vi "ObslugaPieca.vi"() -> ()   [LabVIEW 2012]
doc: "Use this template to build a user interface event handler design pattern. Use this pattern for dialog boxes and other user interfaces. You also can create and execute user-defined events that the VI can handle the same way as user interface events."
uses:
  MachineStatesEnum.ctl
  <vilib>/Utility/file.llb/Write To Spreadsheet File (I64).vi
  <vilib>/Utility/file.llb/Write To Spreadsheet File (string).vi
  <vilib>/Utility/file.llb/Read From Spreadsheet File (string).vi
panel:
  out "wyniki":i16[](array[numeric])
  in  "doStop":bool
  out "Data loaded":bool=TRUE
  in  "SendTelegramDone":bool=TRUE
  in  "Next state":T1=enum."Initialized"
  in  "ProgramStopped":bool=TRUE
  out "Telegrams array":string[](array[string])
  in  "Tab Control":T2(tab)
  in  "Initialize":bool
  in  "VISA resource name":refnum<visa-resource-name>="COM10"
  in  "Load configuration":bool
  in  "Save configuration":bool
  in  "Configure":bool
  out "Telegram1":string
  in  "Temperatura 1":u16 max=400 step=1 format="%03d"
  in  "Godzin 1":u16 max=24 step=1 format="%02d"
  in  "Minut 1":u16 max=59 step=1 format="%02d"
  in  "Sekund 1":u16 max=59 step=1 format="%02d"
  out "Telegram2":string
  in  "Temperatura 2":u16 max=400 step=1 format="%03d"
  in  "Godzin 2":u16 max=24 step=1 format="%02d"
  in  "Minut 2":u16 max=59 step=1 format="%02d"
  in  "Sekund 2":u16 max=59 step=1 format="%02d"
  out "Telegram3":string
  in  "Temperatura 3":u16 max=400 step=1 format="%03d"
  in  "Godzin 3":u16 max=24 step=1 format="%02d"
  in  "Minut 3":u16 max=59 step=1 format="%02d"
  in  "Sekund 3":u16 max=59 step=1 format="%02d"
  in  "Temperatura 6":u16 max=400 step=1 format="%03d"
  in  "Godzin 6":u16 max=24 step=1 format="%02d"
  in  "Minut 6":u16 max=59 step=1 format="%02d"
  in  "Sekund 6":u16 max=59 step=1 format="%02d"
  out "Telegram4":string
  in  "Temperatura 4":u16 max=400 step=1 format="%03d"
  in  "Godzin 4":u16 max=24 step=1 format="%02d"
  in  "Minut 4":u16 max=59 step=1 format="%02d"
  in  "Sekund 4":u16 max=59 step=1 format="%02d"
  in  "Temperatura 5":u16 max=400 step=1 format="%03d"
  in  "Godzin 5":u16 max=24 step=1 format="%02d"
  in  "Minut 5":u16 max=59 step=1 format="%02d"
  in  "Sekund 5":u16 max=59 step=1 format="%02d"
  out "Telegram6":string
  out "Telegram5":string
  out "Wykres zmian temperatury":i16[](graph)
  out "Stan pieca":string
  out "Numer  zadanego programu":string
  in  "Stop":bool
  in  "Port Errors":errorcluster
  out "OdpowiedŸ pieca":string
  in  "Odbiorcy":string
  in  "Wyœlij e-mail przy koñcu":bool
  # "Kolejne programy (nie obowi¹zkowe)"
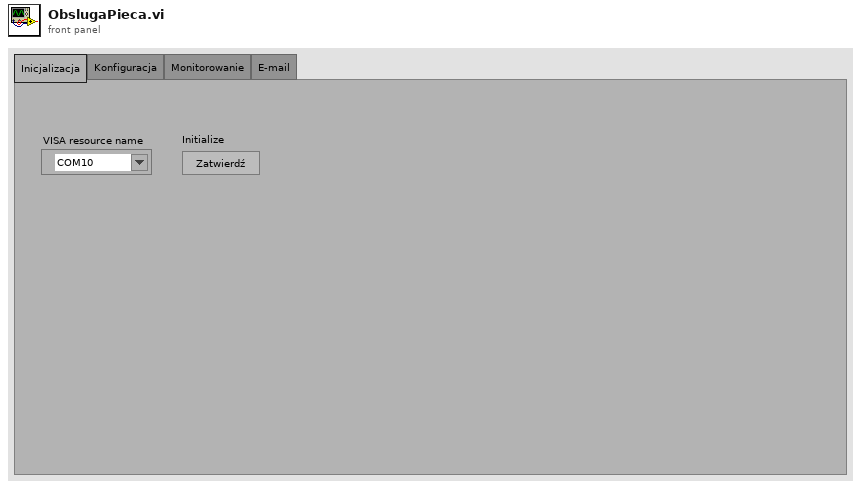
[diagram p1: front panel]
types:
  T1 = typedef "MachineStatesEnum.ctl" = enum16{"StartState", "Initialized", "Configured", "Monitoring", "Ended", "Stopped", "ErrorState"}
  T2 = enum32{"Inicjalizacja", "Konfiguracja", "Monitorowanie", "E-mail"}
  T3 = enum32{"Inicjalizacja", "Konfiguracja", "Monitorowanie"}
  T4 = enum8{"Enabled", "Disabled", "Disabled and Grayed Out"}
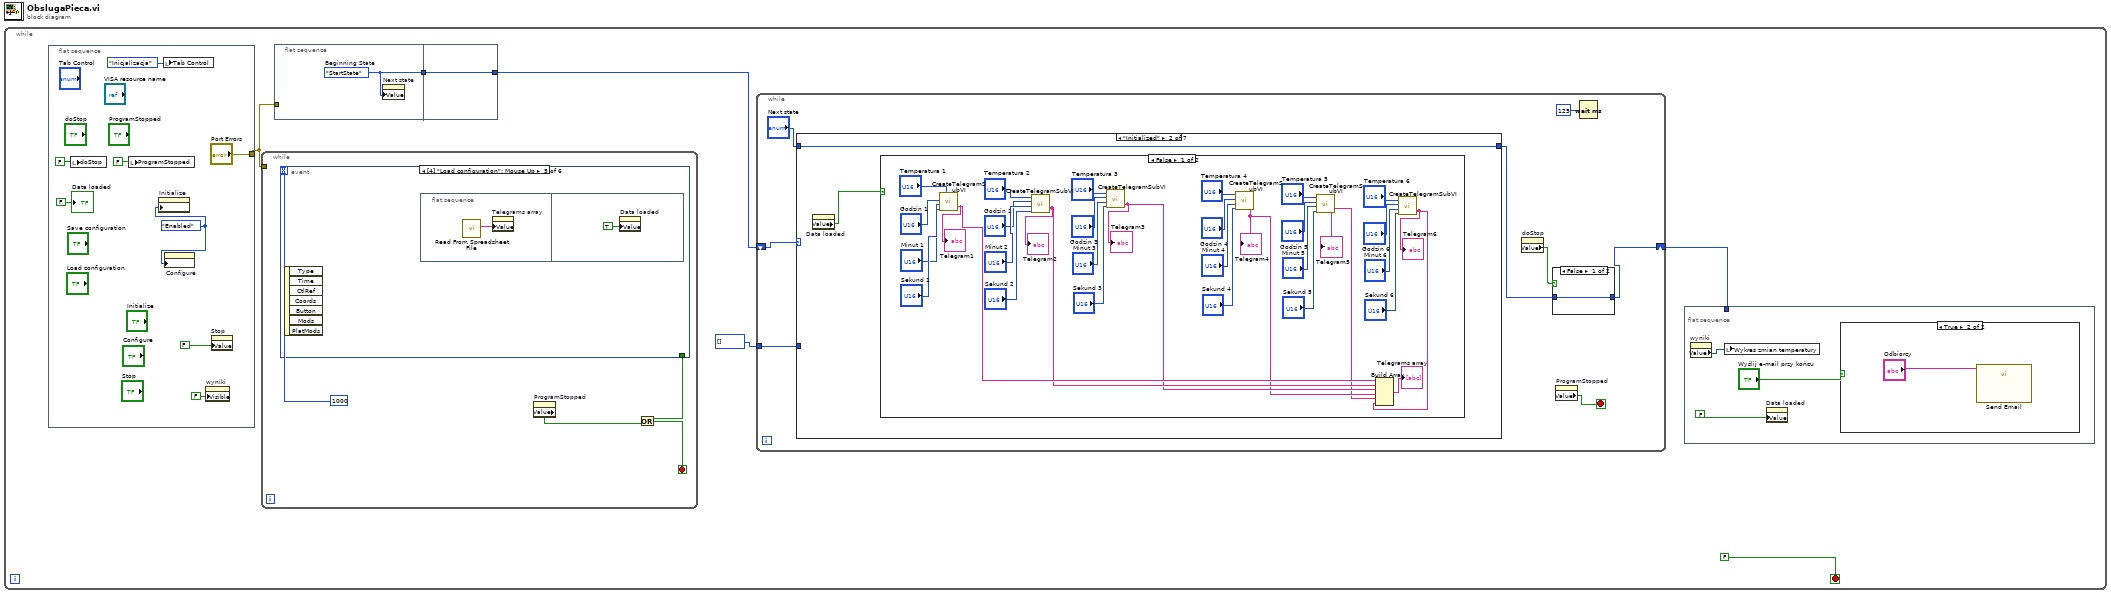
[diagram p0: block diagram]
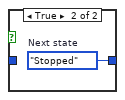
[diagram p3: hidden frame]
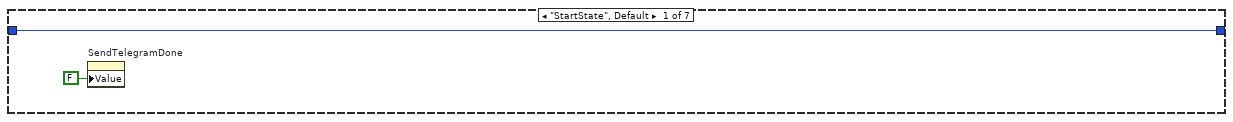
[diagram p4: hidden frame]
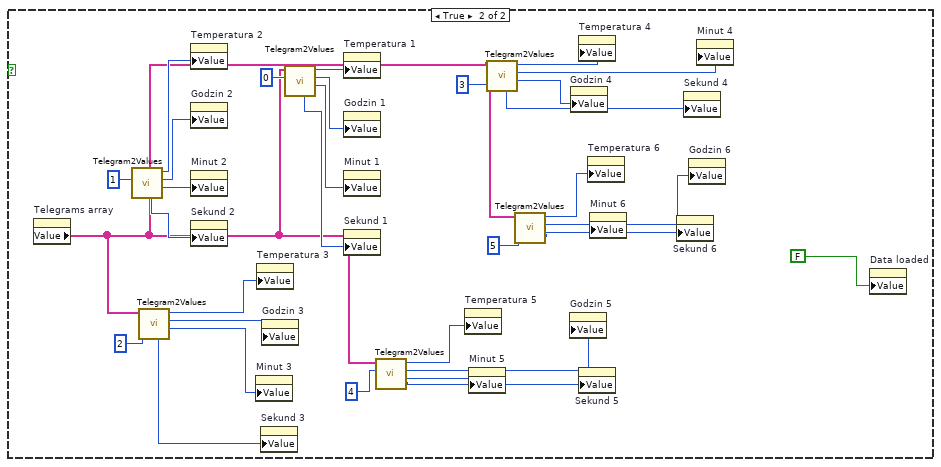
[diagram p5: hidden frame]
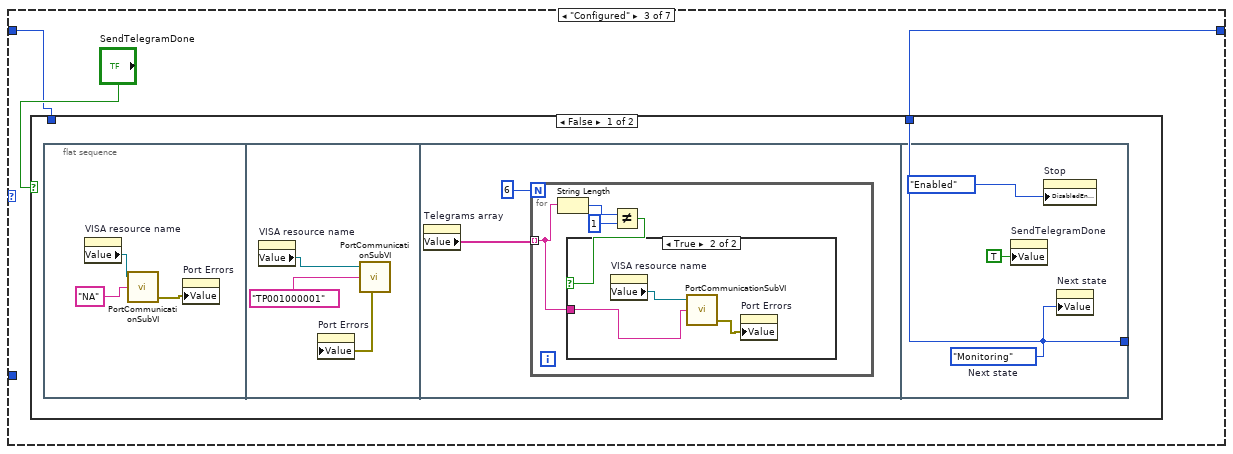
[diagram p6: hidden frame]
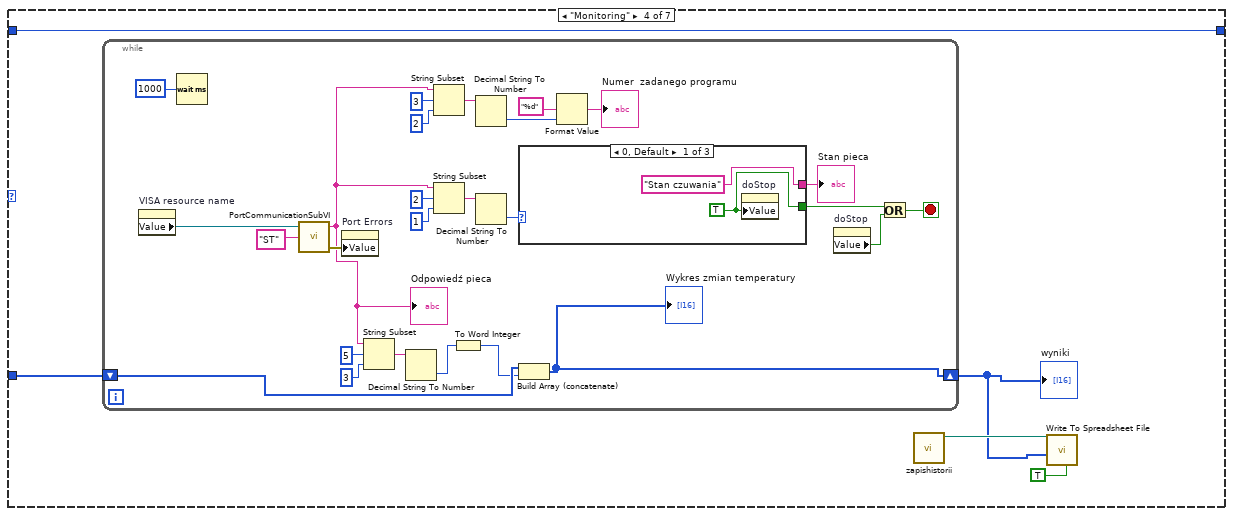
[diagram p9: hidden frame]
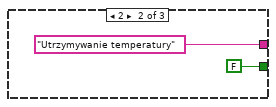
[diagram p10: hidden frame]
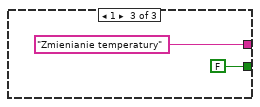
[diagram p11: hidden frame]
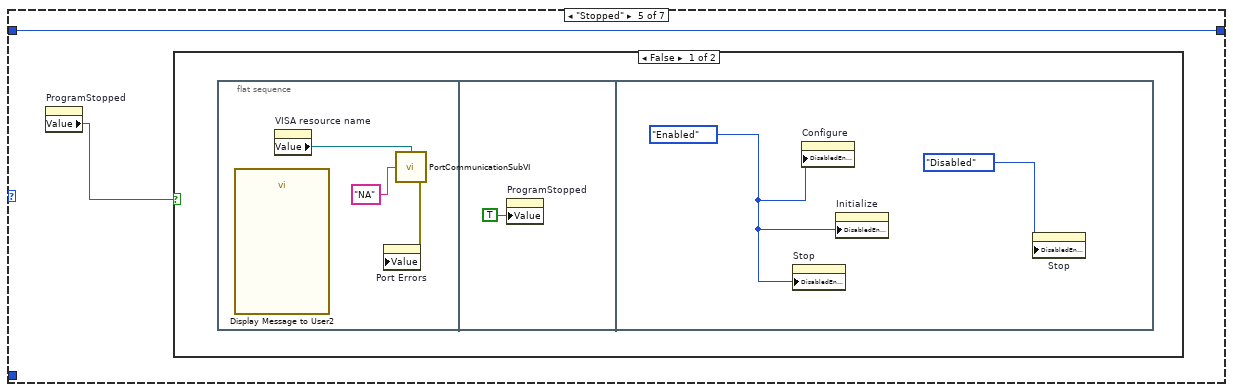
[diagram p12: hidden frame]
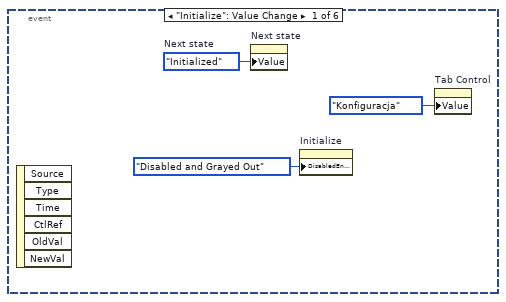
[diagram p16: hidden frame]
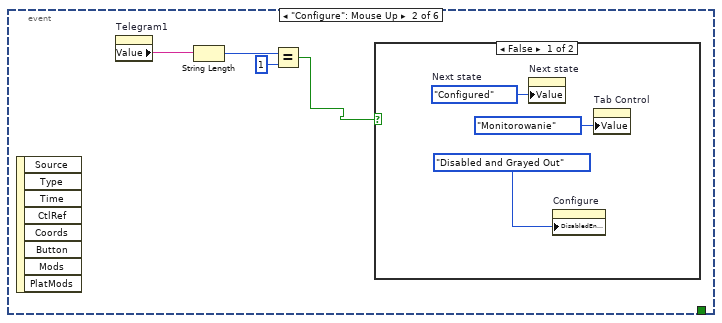
[diagram p17: hidden frame]
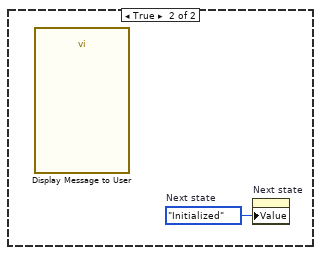
[diagram p18: hidden frame]
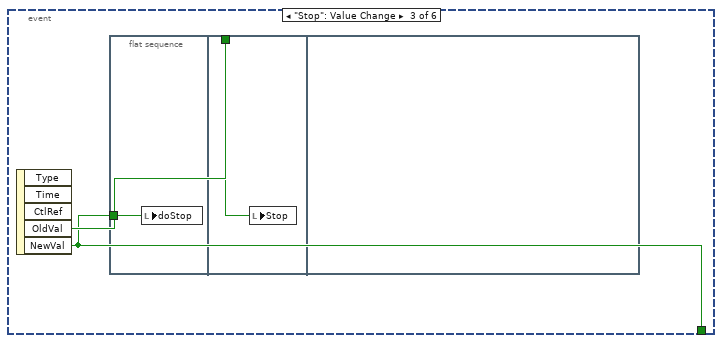
[diagram p19: hidden frame]
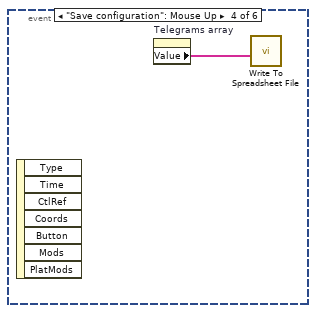
[diagram p20: hidden frame]
diagram:
  n1 = while {
    stop <- FALSE stop-if-true
    n2 = flat-sequence {
      tunnel: ["Port Errors"] -> w4
      frame #0 {
        w13 = T4."Enabled" ("Disabled")
        n3 = local write "doStop"(FALSE ("doStop")) -> ()
        n4 = local write "ProgramStopped"(FALSE ("ProgramStopped")) -> ()
        n5 = property on="Initialize" class="Bool"("DisabledEnum"=w13) -> ()  [unwired: 2 in, 2 out]
        n6 = local write "Tab Control"(T3."Inicjalizacja" ("Tab Control")) -> ()
        n7 = property on="Configure" class="Bool"("DisabledEnum"=w13) -> ()  [unwired: 2 in, 2 out]
        n8 = property on="wyniki" class="Arr (strict)"("Visible"=FALSE) -> ()  [unwired: 2 in, 2 out]
        n9 = property on="Stop" class="Bool (strict)"("Value"=FALSE) -> ()  [unwired: 2 in, 2 out]
        "Data loaded" <- FALSE ("Data loaded")
      }
    }
    n10 = while {
      tunnel: w4 -> [_]
      stop <- w169 stop-if-true
      n11 = event shown="[4] \"Load configuration\": Mouse Up" {
        selector: _ -> [_ _ _ _ _ _]
        dyn-events: _ -> [_ _ _ _ _ _]
        timeout: 1000 -> [_ _ _ _ _ _]
        tunnel: [_ _ w183 _ _ _] -> w171
        event "Initialize": Value Change {
          w173 = MachineStatesEnum."Initialized"  # Next state
          n12 = event-data() -> ()  [unwired: 1 in, 6 out]
          n13 = property on="Next state" class="Enum (strict)"("Value"=w173) -> ()  [unwired: 2 in, 2 out]
          n14 = property on="Initialize" class="Bool"("DisabledEnum"=T4."Disabled and Grayed Out" ("Disabled")) -> ()  [unwired: 2 in, 2 out]
          n15 = property on="Tab Control" class="TabCtl (strict)"("Value"=T3."Konfiguracja" ("Tab Control")) -> ()  [unwired: 2 in, 2 out]
        }
        event "Configure": Mouse Up {
          n16 = event-data() -> ()  [unwired: 1 in, 8 out]
          n17 = property on="Telegram1" class="Str"() -> ("Value"=w176:string)  [unwired: 2 in, 2 out]
          n18 = String Length(string=w176) -> (length=w178:i32)
          n19 = Equal?(x=w178, y=1) -> (x = y?=w175:bool)
          n20 = case shown="False" w175 {
            frame False {
              w180 = MachineStatesEnum."Configured"  # Next state
              n21 = property on="Next state" class="Enum (strict)"("Value"=w180) -> ()  [unwired: 2 in, 2 out]
              n22 = property on="Configure" class="Bool"("DisabledEnum"=T4."Disabled and Grayed Out" ("Disabled")) -> ()  [unwired: 2 in, 2 out]
              n23 = property on="Tab Control" class="TabCtl (strict)"("Value"=T3."Monitorowanie" ("Tab Control")) -> ()  [unwired: 2 in, 2 out]
            }
            frame True {
              w182 = MachineStatesEnum."Initialized"  # Next state
              n24 = call "Display Message to User"() -> ()  [unwired: 10 in, 2 out]
              n25 = property on="Next state" class="Enum (strict)"("Value"=w182) -> ()  [unwired: 2 in, 2 out]
            }
          }
        }
        event "Stop": Value Change {
          n26 = event-data() -> ("OldVal"=w184:bool, "NewVal"=w183:bool)  [unwired: 1 in, 3 out]
          n27 = flat-sequence {
            tunnel: w183 -> [w185]
            tunnel: w184 -> [w186]
            frame #0 {
              n28 = local write "doStop"(w185) -> ()
            }
            frame #1 {
              n29 = local write "Stop"(w186) -> ()
            }
            frame #2 {
            }
          }
        }
        event "Save configuration": Mouse Up {
          n30 = event-data() -> ()  [unwired: 1 in, 7 out]
          n31 = property on="Telegrams array" class="Arr (strict)"() -> ("Value"=w187:string[])  [unwired: 2 in, 2 out]
          n32 = call-poly <vilib>:"Write To Spreadsheet File.vi"("1D data"=w187) -> ()  [unwired: 7 in, 1 out]
        }
        event "Load configuration": Mouse Up {
          n33 = event-data() -> ()  [unwired: 1 in, 7 out]
          n34 = flat-sequence {
            frame #0 {
              n35 = call-poly <vilib>:"Read From Spreadsheet File.vi"() -> ("first row"=w188:string[])  [unwired: 7 in, 4 out]
              n36 = property on="Telegrams array" class="Arr (strict)"("Value"=w188) -> ()  [unwired: 2 in, 2 out]
            }
            frame #1 {
              n37 = property on="Data loaded" class="Bool (strict)"("Value"=TRUE) -> ()  [unwired: 2 in, 2 out]
            }
          }
        }
        event Timeout {
          n38 = event-data() -> ()  [unwired: 1 in, 3 out]
        }
      }
      n39 = property on="ProgramStopped" class="Bool (strict)"() -> ("Value"=w170:bool)  [unwired: 2 in, 2 out]
      n40 = Or(x=w171, y=w170) -> (x .or. y?=w169:bool)
    }
    n41 = flat-sequence {
      tunnel: [w19] -> w6
      tunnel: w4 -> [_]
      tunnel: [w20] -> w5
      tunnel: w6 -> [w20]
      frame #0 {
        w19 = MachineStatesEnum."StartState"  # Beginning State
        n42 = property on="Next state" class="Enum (strict)"("Value"=w19) -> ()  [unwired: 2 in, 2 out]
      }
      frame #1 {
      }
    }
    n43 = while {
      shift-right: [w23] -> w2
      shift-left: w5 -> [w27]
      tunnel: i16[] [] -> [w21]
      stop <- w25 stop-if-true
      n44 = case shown="\"Initialized\"" w27 {
        selector: w27 -> [_ _ _ _ _ w166 w167]
        tunnel: [w32 w34 w98 w125 w159 w166 w167] -> w24
        tunnel: "Next state" -> [w32 w34 w99 w125 w159 _ _]
        tunnel: w21 -> [_ _ _ w124 _ _ _]
        frame "StartState", Default {
          n45 = property on="SendTelegramDone" class="Bool (strict)"("Value"=FALSE ("SendTelegramDone")) -> ()  [unwired: 2 in, 2 out]
        }
        frame "Initialized" {
          n46 = property on="Data loaded" class="Bool (strict)"() -> ("Value"=w33:bool)  [unwired: 2 in, 2 out]
          n47 = case shown="False" w33 {
            frame False {
              n48 = call "CreateTelegramSubVI.vi"("seconds"="Sekund 1", "minutes"="Minut 1", "hours"="Godzin 1", "temperature"="Temperatura 1") -> ("tempTelegram"=w41:string)  [unwired: 1 in]
              "Telegram1" <- w41
              n49 = call "CreateTelegramSubVI.vi"("seconds"="Sekund 2", "minutes"="Minut 2", "hours"="Godzin 2", "temperature"="Temperatura 2") -> ("tempTelegram"=w40:string)  [unwired: 1 in]
              "Telegram2" <- w40
              n50 = call "CreateTelegramSubVI.vi"("seconds"="Sekund 3", "minutes"="Minut 3", "hours"="Godzin 3", "temperature"="Temperatura 3") -> ("tempTelegram"=w39:string)  [unwired: 1 in]
              "Telegram3" <- w39
              n51 = call "CreateTelegramSubVI.vi"("seconds"="Sekund 4", "minutes"="Minut 4", "hours"="Godzin 4", "temperature"="Temperatura 4") -> ("tempTelegram"=w38:string)  [unwired: 1 in]
              "Telegram4" <- w38
              n52 = call "CreateTelegramSubVI.vi"("seconds"="Sekund 5", "minutes"="Minut 5", "hours"="Godzin 5", "temperature"="Temperatura 5") -> ("tempTelegram"=w37:string)  [unwired: 1 in]
              "Telegram5" <- w37
              n53 = call "CreateTelegramSubVI.vi"("seconds"="Sekund 6", "minutes"="Minut 6", "hours"="Godzin 6", "temperature"="Temperatura 6") -> ("tempTelegram"=w36:string)  [unwired: 1 in]
              "Telegram6" <- w36
              n54 = Build Array(w41, w40, w39, w38, w37, w36) -> (→"Telegrams array":string[])
            }
            frame True {
              n55 = property on="Telegrams array" class="Arr (strict)"() -> ("Value"=w87:string[])  [unwired: 2 in, 2 out]
              n56 = call "Telegram2Values.vi"("index"=1, "Value"=w87) -> ("Numeric 2"=w89:u16, "Numeric 3"=w90:u16, "Numeric 4"=w91:u16, "Numeric"=w88:u16)  [unwired: 6 in]
              n57 = call "Telegram2Values.vi"("index"=2, "Value"=w87) -> ("Numeric 2"=w80:u16, "Numeric 3"=w81:u16, "Numeric 4"=w82:u16, "Numeric"=w79:u16)  [unwired: 6 in]
              n58 = property on="Temperatura 2" class="DigNum (strict)"("Value"=w91) -> ()  [unwired: 2 in, 2 out]
              n59 = property on="Godzin 2" class="DigNum (strict)"("Value"=w90) -> ()  [unwired: 2 in, 2 out]
              n60 = property on="Minut 2" class="DigNum (strict)"("Value"=w89) -> ()  [unwired: 2 in, 2 out]
              n61 = property on="Sekund 2" class="DigNum (strict)"("Value"=w88) -> ()  [unwired: 2 in, 2 out]
              n62 = property on="Minut 3" class="DigNum (strict)"("Value"=w80) -> ()  [unwired: 2 in, 2 out]
              n63 = property on="Temperatura 3" class="DigNum (strict)"("Value"=w82) -> ()  [unwired: 2 in, 2 out]
              n64 = property on="Sekund 3" class="DigNum (strict)"("Value"=w79) -> ()  [unwired: 2 in, 2 out]
              n65 = property on="Godzin 3" class="DigNum (strict)"("Value"=w81) -> ()  [unwired: 2 in, 2 out]
              n66 = call "Telegram2Values.vi"("index"=0, "Value"=w87) -> ("Numeric 2"=w94:u16, "Numeric 3"=w96:u16, "Numeric 4"=w97:u16, "Numeric"=w93:u16)  [unwired: 6 in]
              n67 = property on="Temperatura 1" class="DigNum (strict)"("Value"=w97) -> ()  [unwired: 2 in, 2 out]
              n68 = property on="Godzin 1" class="DigNum (strict)"("Value"=w96) -> ()  [unwired: 2 in, 2 out]
              n69 = property on="Minut 1" class="DigNum (strict)"("Value"=w94) -> ()  [unwired: 2 in, 2 out]
              n70 = property on="Sekund 1" class="DigNum (strict)"("Value"=w93) -> ()  [unwired: 2 in, 2 out]
              n71 = call "Telegram2Values.vi"("index"=4, "Value"=w87) -> ("Numeric 2"=w72:u16, "Numeric 3"=w73:u16, "Numeric 4"=w74:u16, "Numeric"=w71:u16)  [unwired: 6 in]
              n72 = property on="Temperatura 5" class="DigNum (strict)"("Value"=w74) -> ()  [unwired: 2 in, 2 out]
              n73 = property on="Minut 5" class="DigNum (strict)"("Value"=w72) -> ()  [unwired: 2 in, 2 out]
              n74 = call "Telegram2Values.vi"("index"=3, "Value"=w87) -> ("Numeric 2"=w76:u16, "Numeric 3"=w77:u16, "Numeric 4"=w78:u16, "Numeric"=w75:u16)  [unwired: 6 in]
              n75 = call "Telegram2Values.vi"("index"=5, "Value"=w87) -> ("Numeric 2"=w68:u16, "Numeric 3"=w69:u16, "Numeric 4"=w70:u16, "Numeric"=w67:u16)  [unwired: 6 in]
              n76 = property on="Godzin 5" class="DigNum (strict)"("Value"=w73) -> ()  [unwired: 2 in, 2 out]
              n77 = property on="Godzin 4" class="DigNum (strict)"("Value"=w76) -> ()  [unwired: 2 in, 2 out]
              n78 = property on="Temperatura 4" class="DigNum (strict)"("Value"=w78) -> ()  [unwired: 2 in, 2 out]
              n79 = property on="Sekund 5" class="DigNum (strict)"("Value"=w71) -> ()  [unwired: 2 in, 2 out]
              n80 = property on="Temperatura 6" class="DigNum (strict)"("Value"=w70) -> ()  [unwired: 2 in, 2 out]
              n81 = property on="Minut 6" class="DigNum (strict)"("Value"=w68) -> ()  [unwired: 2 in, 2 out]
              n82 = property on="Sekund 6" class="DigNum (strict)"("Value"=w67) -> ()  [unwired: 2 in, 2 out]
              n83 = property on="Sekund 4" class="DigNum (strict)"("Value"=w75) -> ()  [unwired: 2 in, 2 out]
              n84 = property on="Godzin 6" class="DigNum (strict)"("Value"=w69) -> ()  [unwired: 2 in, 2 out]
              n85 = property on="Minut 4" class="DigNum (strict)"("Value"=w77) -> ()  [unwired: 2 in, 2 out]
              n86 = property on="Data loaded" class="Bool (strict)"("Value"=FALSE) -> ()  [unwired: 2 in, 2 out]
            }
          }
        }
        frame "Configured" {
          n87 = case shown="False" "SendTelegramDone" {
            tunnel: w99 -> [_ w120]
            tunnel: [w101 w120] -> w98
            frame False {
              n88 = flat-sequence {
                tunnel: [w118] -> w101
                frame #0 {
                  n89 = property on="VISA resource name" class="VISAName"() -> ("Value"=w102:refnum<visa-resource-name>)  [unwired: 2 in, 2 out]
                  n90 = call "PortCommunicationSubVI.vi"("Value"="NA", "VISA Refnum in"=w102) -> ("error out"=w103:errorcluster)  [unwired: 2 in, 1 out]
                  n91 = property on="Port Errors" class="Clust (strict)"("Value"=w103) -> ()  [unwired: 2 in, 2 out]
                }
                frame #1 {
                  n92 = property on="VISA resource name" class="VISAName"() -> ("Value"=w107:refnum<visa-resource-name>)  [unwired: 2 in, 2 out]
                  n93 = call "PortCommunicationSubVI.vi"("Value"="TP001000001", "VISA Refnum in"=w107) -> ("error out"=w106:errorcluster)  [unwired: 2 in, 1 out]
                  n94 = property on="Port Errors" class="Clust (strict)"("Value"=w106) -> ()  [unwired: 2 in, 2 out]
                }
                frame #2 {
                  n95 = property on="Telegrams array" class="Arr (strict)"() -> ("Value"=w108:string[])  [unwired: 2 in, 2 out]
                  n96 = for {
                    N: 6 -> [_]
                    tunnel: w108 -> [w110] mode=indexing
                    n97 = String Length(string=w110) -> (length=w111:i32)
                    n98 = Not Equal?(x=w111, y=1) -> (x != y?=w113:bool)
                    n99 = case shown="True" w113 {
                      tunnel: w110 -> [_ w115]
                      frame False {
                      }
                      frame True {
                        n100 = property on="VISA resource name" class="VISAName"() -> ("Value"=w116:refnum<visa-resource-name>)  [unwired: 2 in, 2 out]
                        n101 = call "PortCommunicationSubVI.vi"("Value"=w115, "VISA Refnum in"=w116) -> ("error out"=w114:errorcluster)  [unwired: 2 in, 1 out]
                        n102 = property on="Port Errors" class="Clust (strict)"("Value"=w114) -> ()  [unwired: 2 in, 2 out]
                      }
                    }
                  }
                }
                frame #3 {
                  w118 = MachineStatesEnum."Monitoring"  # Next state
                  n103 = property on="SendTelegramDone" class="Bool (strict)"("Value"=TRUE ("SendTelegramDone")) -> ()  [unwired: 2 in, 2 out]
                  n104 = property on="Stop" class="Bool (strict)"("DisabledEnum"=T4."Enabled" ("Disabled")) -> ()  [unwired: 2 in, 2 out]
                  n105 = property on="Next state" class="Enum (strict)"("Value"=w118) -> ()  [unwired: 2 in, 2 out]
                }
              }
            }
            frame True {
            }
          }
        }
        frame "Monitoring" {
          n106 = while {
            shift-right: [w126] -> w122
            shift-left: w124 -> [w129]
            stop <- w132 stop-if-true
            n107 = property on="VISA resource name" class="VISAName"() -> ("Value"=w137:refnum<visa-resource-name>)  [unwired: 2 in, 2 out]
            n108 = Wait (ms)(milliseconds to wait=u32 1000) -> ()  [unwired: 1 out]
            n109 = call "PortCommunicationSubVI.vi"("Value"="ST", "VISA Refnum in"=w137) -> ("error out"=w135:errorcluster, "read buffer"=w134:string)  [unwired: 2 in]
            "OdpowiedŸ pieca" <- w134
            n110 = property on="Port Errors" class="Clust (strict)"("Value"=w135) -> ()  [unwired: 2 in, 2 out]
            n111 = String Subset(string=w134, offset (0)=5, length (rest)=3 ("length (rest)")) -> (substring=w148:string)
            n112 = Decimal String To Number(string=w148) -> (number=w128:i32)  [unwired: 2 in, 1 out]
            n113 = String Subset(string=w134, offset (0)=3, length (rest)=2 ("length (rest)")) -> (substring=w140:string)
            n114 = String Subset(string=w134, offset (0)=2, length (rest)=1 ("length (rest)")) -> (substring=w145:string)
            n115 = To Word Integer(number=w128) -> (16bit integer=w127:i16)
            n116 = Decimal String To Number(string=w140) -> (number=w131:i32)  [unwired: 2 in, 1 out]
            n117 = Decimal String To Number(string=w145) -> (number=w143:i32)  [unwired: 2 in, 1 out]
            n118 = case shown="0, Default" w143 {
              tunnel: ["Stan czuwania" ("Stan pieca") "Utrzymywanie temperatury" ("Stan pieca") "Zmienianie temperatury" ("Stan pieca")] -> w144
              tunnel: [w152 FALSE ("y") FALSE ("y")] -> w133
              frame 0, Default {
                w152 = TRUE ("y")
                n119 = property on="doStop" class="Bool (strict)"("Value"=w152) -> ()  [unwired: 2 in, 2 out]
              }
              frame 2 {
              }
              frame 1 {
              }
            }
            "Stan pieca" <- w144
            n120 = Build Array (concatenate)(w129, w127) -> (w126:i16[])
            "Wykres zmian temperatury" <- w126
            n121 = Format Value(format string="%d", value (0)=w131) -> (output string=→"Numer  zadanego programu":string)  [unwired: 1 in]
            n122 = property on="doStop" class="Bool (strict)"() -> ("Value"=w130:bool)  [unwired: 2 in, 2 out]
            n123 = Or(x=w133, y=w130) -> (x .or. y?=w132:bool)
          }
          "wyniki" <- w122
          n124 = call "zapishistorii.vi"() -> ("appended path"=w123:path)  [unwired: 11 in]
          n125 = call-poly <vilib>:"Write To Spreadsheet File.vi"("transpose? (no:F)"=TRUE, "1D data"=w122, "file path (dialog if empty)"=w123) -> ()  [unwired: 5 in, 1 out]
        }
        frame "Stopped" {
          n126 = property on="ProgramStopped" class="Bool (strict)"() -> ("Value"=w158:bool)  [unwired: 2 in, 2 out]
          n127 = case shown="False" w158 {
            frame False {
              n128 = flat-sequence {
                frame #0 {
                  n129 = call "Display Message to User2"() -> ()  [unwired: 10 in, 2 out]
                  n130 = property on="VISA resource name" class="VISAName"() -> ("Value"=w162:refnum<visa-resource-name>)  [unwired: 2 in, 2 out]
                  n131 = call "PortCommunicationSubVI.vi"("Value"="NA", "VISA Refnum in"=w162) -> ("error out"=w161:errorcluster)  [unwired: 2 in, 1 out]
                  n132 = property on="Port Errors" class="Clust (strict)"("Value"=w161) -> ()  [unwired: 2 in, 2 out]
                }
                frame #1 {
                  n133 = property on="ProgramStopped" class="Bool (strict)"("Value"=TRUE ("ProgramStopped")) -> ()  [unwired: 2 in, 2 out]
                }
                frame #2 {
                  w165 = T4."Enabled" ("Disabled")
                  n134 = property on="Stop" class="Bool (strict)"("DisabledEnum"=w165) -> ()  [unwired: 2 in, 2 out]
                  n135 = property on="Configure" class="Bool"("DisabledEnum"=w165) -> ()  [unwired: 2 in, 2 out]
                  n136 = property on="Initialize" class="Bool"("DisabledEnum"=w165) -> ()  [unwired: 2 in, 2 out]
                  n137 = property on="Stop" class="Bool (strict)"("DisabledEnum"=T4."Disabled" ("Disabled")) -> ()  [unwired: 2 in, 2 out]
                }
              }
            }
            frame True {
            }
          }
        }
        frame "Ended" {
        }
        frame "ErrorState" {
        }
      }
      n138 = property on="doStop" class="Bool (strict)"() -> ("Value"=w22:bool)  [unwired: 2 in, 2 out]
      n139 = case shown="False" w22 {
        tunnel: w24 -> [w29 _]
        tunnel: [w29 w30] -> w23
        frame False {
        }
        frame True {
          w30 = MachineStatesEnum."Stopped"  # Next state
        }
      }
      n140 = property on="ProgramStopped" class="Bool (strict)"() -> ("Value"=w25:bool)  [unwired: 2 in, 2 out]
      n141 = Wait (ms)(milliseconds to wait=u32 125) -> ()  [unwired: 1 out]
    }
    n142 = flat-sequence {
      tunnel: w2 -> [_]
      frame #0 {
        n143 = property on="wyniki" class="Arr (strict)"() -> ("Value"=w9:i16[])  [unwired: 2 in, 2 out]
        n144 = local write "Wykres zmian temperatury"(w9) -> ()
        n145 = property on="Data loaded" class="Bool (strict)"("Value"=FALSE) -> ()  [unwired: 2 in, 2 out]
        n146 = case shown="True" "Wyœlij e-mail przy koñcu" {
          frame False {
          }
          frame True {
            n147 = call "Send Email"("Recipients"="Odbiorcy") -> ()  [unwired: 10 in, 1 out]
          }
        }
      }
    }
  }
